vi "sv_Increment_AO Freq Index.vi"(4 "AO block Size":i32, 6 "AO freq index":i32, 7 "frequency\n to generate [Hz]":dbl format="%.2f", 8 "amplitude list":dbl[](array[numeric]) format="%.2f", 9 "frequency list":dbl[](array[numeric]) format="%.2f", 10 "repeat":enum16{"off", "on"}(ring), 11 "write index - freq stop index":i32) -> (2 "freq":T1={"samples [current]"=128, "current amplitude"=0.0, "current frequency [Hz]"=0.0, "samples [next]"=128, "next amplitude"=0.0, "next frequency (Hz)"=0.0} {"next frequency (Hz)" format="%.2f"; "next amplitude" format="%.2f"; "current amplitude" format="%.2f"; "current frequency [Hz]" format="%.2f"}, 3 "AO freq index":i32, 5 "case":T2(ring))   [LabVIEW 2017, in "SoundVib_SweptSine.lvlib"]
uses:
  <vilib>/addons/Sound and Vibration/svt_Swept Sine/SoundVib_SweptSine.lvlib
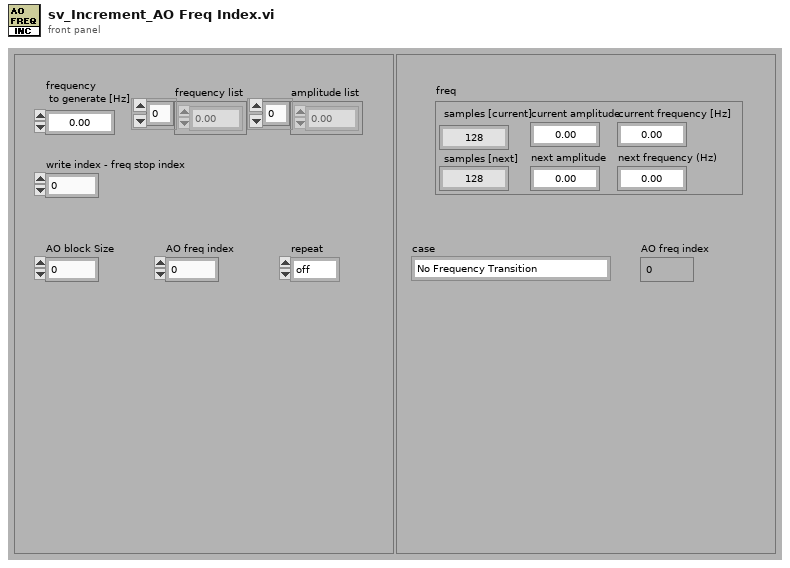
[diagram p1: front panel]
types:
  T1 = cluster{"samples [current]":i32, "current amplitude":dbl, "current frequency [Hz]":dbl, "samples [next]":i32, "next amplitude":dbl, "next frequency (Hz)":dbl}
  T2 = enum16{"No Frequency Transition", "Transition to Next Frequency", "Transition to DC (last block)"}
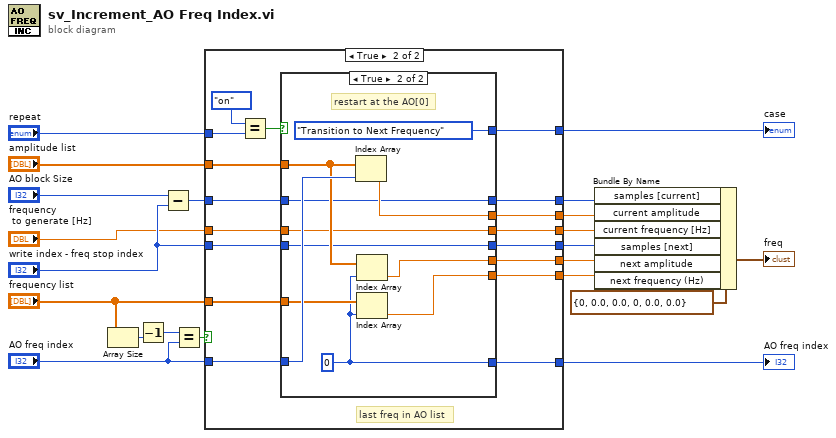
[diagram p0: block diagram]
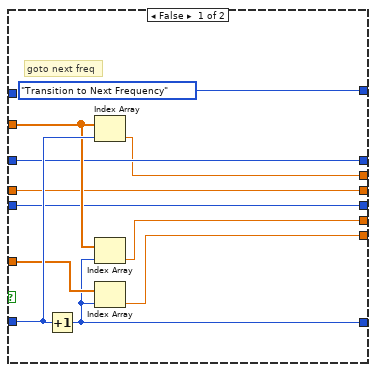
[diagram p2: hidden frame]
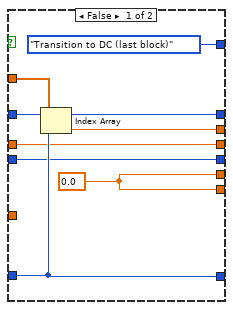
[diagram p3: hidden frame]
diagram:
  n1 = Array Size(array="frequency list") -> (size(s)=w19:i32)
  n2 = Decrement(x=w19) -> (x-1=w10:i32)
  n3 = Subtract(x="AO block Size", y="write index - freq stop index") -> (x-y=w17:i32)
  n4 = Equal?(x=w10, y="AO freq index") -> (x = y?=w18:bool)
  n5 = case shown="True" w18 {
    tunnel: "AO freq index" -> [w32 w45]
    tunnel: "frequency\n to generate [Hz]" -> [w22 w46]
    tunnel: w17 -> [w27 w47]
    tunnel: "write index - freq stop index" -> [w26 w44]
    tunnel: "frequency list" -> [w31 w43]
    tunnel: [T2."Transition to Next Frequency" ("case") w48] -> w21
    tunnel: "amplitude list" -> [w28 w42]
    tunnel: [w29 w41] -> w12
    tunnel: "repeat" -> [_ w34]
    tunnel: [w27 w38] -> w8
    tunnel: [w23 w39] -> w7
    tunnel: [w26 w37] -> w6
    tunnel: [w25 w36] -> w5
    tunnel: [w24 w35] -> w4
    tunnel: [w22 w40] -> w2
    frame False {
      # "goto next freq"
      n6 = Increment(x=w32) -> (x+1=w29:i32)
      n7 = Index Array(array=w28, index=w32) -> (element=w23:dbl)
      n8 = Index Array(array=w28, index=w29) -> (element=w25:dbl)
      n9 = Index Array(array=w31, index=w29) -> (element=w24:dbl)
    }
    frame True {
      # "last freq in AO list"
      n10 = Equal?(x=enum16{"off", "on"}."on" ("y"), y=w34) -> (x = y?=w49:bool)
      n11 = case shown="True" w49 {
        tunnel: [T2."Transition to DC (last block)" ("case") T2."Transition to Next Frequency" ("case")] -> w48
        tunnel: w47 -> [w53 w61]
        tunnel: w46 -> [w51 w63]
        tunnel: w45 -> [w55 w67]
        tunnel: w44 -> [w52 w60]
        tunnel: w43 -> [_ w66]
        tunnel: w42 -> [w56 w65]
        tunnel: [w55 w64] -> w41
        tunnel: [w51 w63] -> w40
        tunnel: [w54 w62] -> w39
        tunnel: [w53 w61] -> w38
        tunnel: [w52 w60] -> w37
        tunnel: [w50 w59] -> w36
        tunnel: [w50 w58] -> w35
        frame False {
          w50 = 0.0
          n12 = Index Array(array=w56, index=w55) -> (element=w54:dbl)
        }
        frame True {
          w64 = 0 ("frequencies indices.AO freq index")
          # "restart at the AO[0]"
          n13 = Index Array(array=w65, index=w67) -> (element=w62:dbl)
          n14 = Index Array(array=w65, index=w64) -> (element=w59:dbl)
          n15 = Index Array(array=w66, index=w64) -> (element=w58:dbl)
        }
      }
    }
  }
  "case" <- w21
  "AO freq index" <- w12
  n16 = Bundle By Name(cluster=T1 {"samples [current]"=0, "current amplitude"=0.0, "current frequency [Hz]"=0.0, "samples [next]"=0, "next amplitude"=0.0, "next frequency (Hz)"=0.0} ("freq"), "samples [current]"=w8, "current amplitude"=w7, "current frequency [Hz]"=w2, "samples [next]"=w6, "next amplitude"=w5, "next frequency (Hz)"=w4) -> (→"freq":T1)
